vi "Hitrap_DiagnosticBoxGUI.constructor.vi"(0 "name":string, 2 "data in":string, 5 "error in (no error)":errorcluster) -> (14 "i ref out":refnum<vi>, 16 "data out":string, 19 "error out":errorcluster)   [LabVIEW 2014, in "Hitrap_DiagnosticBoxGUI.lvlib"]
doc: "This is the constructor of a class.\n\nLicense Agreement for this software:\n\nCopyright (C)\nGesellschaft für Schwerionenforschung, GSI\nPlanckstr. 1\n64291 Darmstadt\nGermany\n\nContact: D.Beck@gsi.de \n\nThis program is free software; you can redistribute it and/or modify it under the terms of the \nGNU General Public License as published by the Free Software Foundation; either version 2 of \nthe license, or (at your option) any later version.\n\nThis program is distributed in the hope that it will be useful, but WITHOUT ANY WARRANTY; \nwithout even the implied warranty of MERCHANTABILITY or FITNESS FOR A PARTICULAR PURPOSE. See the GNU General License for more details (http://www.gnu.org).\n\nGesellschaft für Schwerionenforschung, GSI\nPlanckstr. 1, 64291 Darmstadt, Germany\nFor all questions and ideas contact: M.Richter@gsi.de, H.Brand@gsi.de or D.Beck@gsi.de.\nLast update: 16-JUN-2004"
uses:
  Hitrap_DiagnosticBoxGUI.lvlib
  CS_Core/CSSystem/CSSystemLib/CSSystemLib.lvlib
  CS_Core/GUIs/GOGUserGUIs/DeviceBaseGUI/DeviceBaseGUI.lvlib
  CS_Core/CSObj/CSObj.lvlib
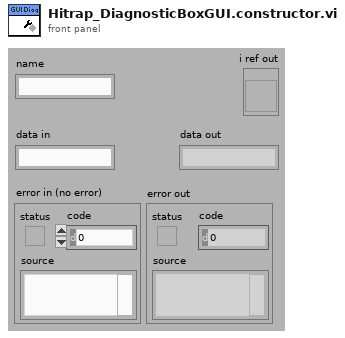
[diagram p1: front panel]
types:
  T1 = enum16{"SetAttribute", "GetAttribute", "CreateAttribute", "DestroyAttribute", "DestroyAllAtributes"}
  T2 = typedef "CSObj.lvlib/CSObj.i attribute.ctl" = cluster{"VI Refnum":refnum<vi>, "Front Panel Ref":refnum<vi>, "semaphore":T3, "date of birth":dbl, "ageID":i32, "systemID":i32, "classID":i32, "conditionID":i32, "DefaultPanelType":u16}
  T3 = typedef "Semaphore RefNum" = refnum<k1>
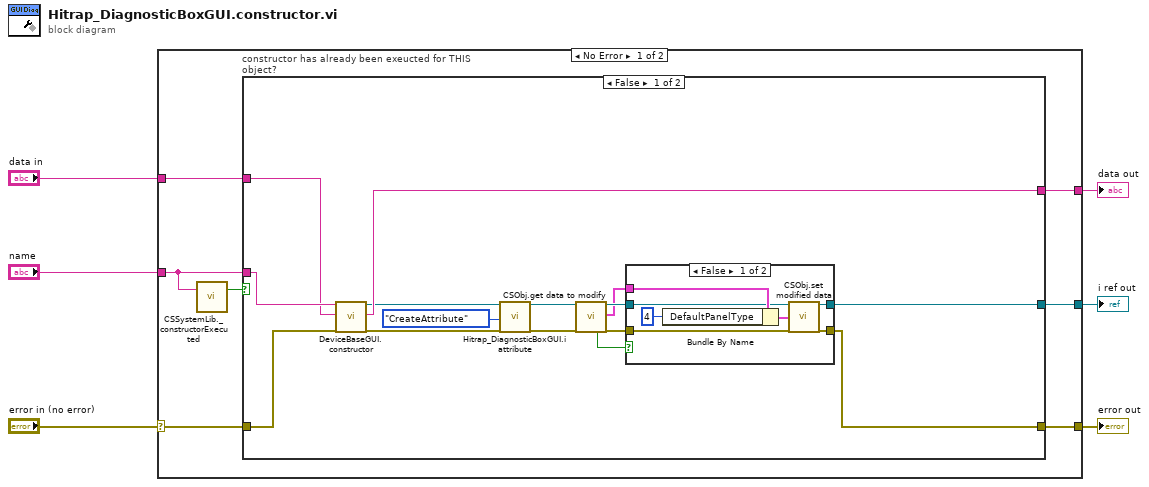
[diagram p0: block diagram]
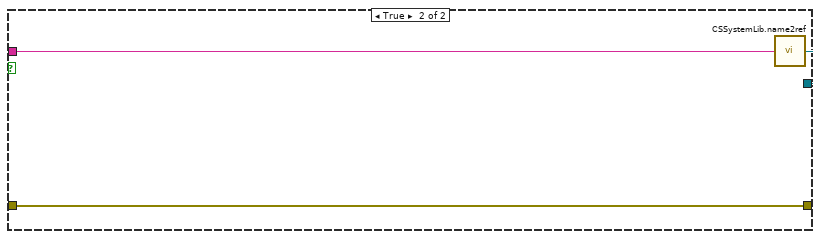
[diagram p3: hidden frame]
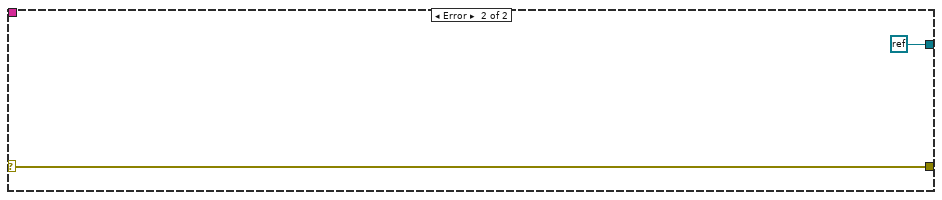
[diagram p4: hidden frame]
diagram:
  n1 = case shown="No Error" "error in (no error)" {
    selector: "error in (no error)" -> [w10 w41]
    tunnel: "data in" -> [w13 _]
    tunnel: "name" -> [w9 _]
    tunnel: [w12 refnum<k0> refnum] -> w4
    tunnel: [w11 w41] -> w3
    tunnel: [w7 _] -> w1
    frame No Error {
      n2 = call "CSSystemLib._constructorExecuted.vi"("name"=w9) -> ("constructor executed?"=w8:bool)  [unwired: 18 in]
      n3 = case "constructor has already been exeucted for THIS object?" shown="False" w8 {
        tunnel: w13 -> [w24 _]
        tunnel: w9 -> [w25 w40]
        tunnel: [w14 w39] -> w12
        tunnel: [w15 w38] -> w11
        tunnel: w10 -> [w27 w38]
        tunnel: [w23 _] -> w7
        frame False {
          n4 = call "DeviceBaseGUI.constructor.vi"("name"=w25, "data in"=w24, "error in (no error)"=w27) -> ("i ref out"=w22:refnum<vi>, "data out"=w23:string, "error out"=w26:errorcluster)  [unwired: 14 in]
          n5 = call "Hitrap_DiagnosticBoxGUI.i attribute.vi"("VI Refnum"=w22, "Action"=T1."CreateAttribute", "error in (no error)"=w26) -> ("VI Refnum out"=w17:refnum<vi>, "error out"=w16:errorcluster)  [unwired: 14 in, 1 out]
          n6 = call "CSObj.get data to modify.vi"("i ref in"=w17, "error in (no error)"=w16) -> ("i ref out"=w20:refnum<vi>, "i attribute"=w18:T2, "timed out"=w21:bool, "error out"=w19:errorcluster)  [unwired: 14 in]
          n7 = case shown="False" w21 {
            tunnel: [w33 w37] -> w14
            tunnel: w20 -> [w34 w37]
            tunnel: [w31 w36] -> w15
            tunnel: w19 -> [w32 w36]
            tunnel: w18 -> [w35 _]
            frame False {
              n8 = Bundle By Name(cluster=w35, "DefaultPanelType"=u16 4) -> (w30:T2)
              n9 = call "CSObj.set modified data.vi"("i ref in"=w34, "i attribute"=w30, "error in (no error)"=w32) -> ("i ref out"=w33:refnum<vi>, "error out"=w31:errorcluster)  [unwired: 15 in]
            }
            frame True {
            }
          }
        }
        frame True {
          n10 = call "CSSystemLib.name2ref.vi"("name"=w40) -> ("obj refnum"=w39:refnum<vi>)
        }
      }
    }
    frame Error {
    }
  }
  "i ref out" <- w4
  "error out" <- w3
  "data out" <- w1
